vi "FTS GetSet Acquisition Option WMtr Cycle Counting.vi"(6 "readWrite":enum16{"read", "write"}(ring), 8 "error in":errorcluster, 9 "cycleCounting":bool, 10 "channel index interferogram":u16, 11 "spectrometerIdx":u16) -> (0 "error out":errorcluster, 1 "cycleCounting read":bool, 3 "FTSLib_status":i32)   [LabVIEW 2010, in "FTSLib.lvlib"]
uses:
  FTSLib.lvlib
  FTSLib.dll
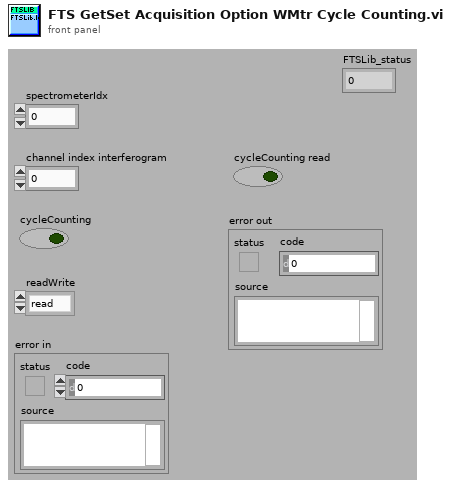
[diagram p1: front panel]
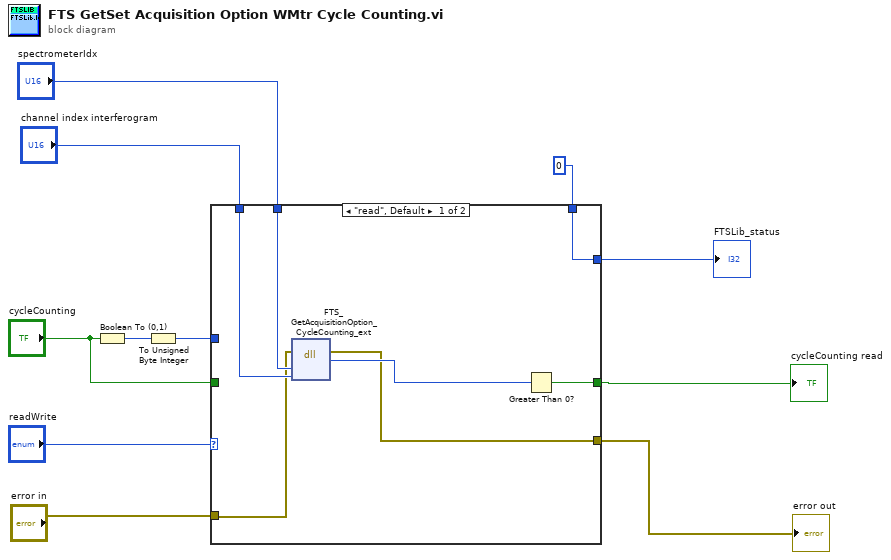
[diagram p0: block diagram]
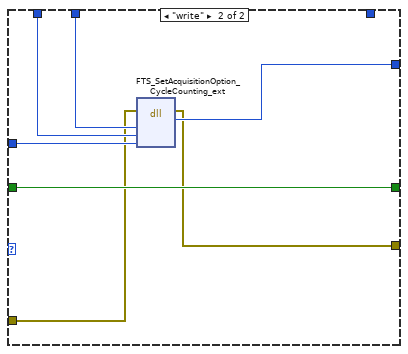
[diagram p2: hidden frame]
diagram:
  n1 = Boolean To (0,1)(Boolean="cycleCounting") -> (0, 1=w6:i16)
  n2 = To Unsigned Byte Integer(number=w6) -> (unsigned 8bit integer=w7:u8)
  n3 = case shown="\"read\", Default" "readWrite" {
    tunnel: "spectrometerIdx" -> [w18 w25]
    tunnel: w7 -> [_ w24]
    tunnel: "error in" -> [w14 w20]
    tunnel: "cycleCounting" -> [_ w23]
    tunnel: [w17 w23] -> w10
    tunnel: [w13 w19] -> w9
    tunnel: "channel index interferogram" -> [w16 w22]
    tunnel: [w12 w21] -> w2
    tunnel: 0 ("return type") -> [w12 _]
    frame "read", Default {
      n4 = dll-call lib="FTSLib.dll" fn="FTS_GetAcquisitionOption_CycleCounting_ext"(error in=w14, "spectrIdx"=w18, "channel"=w16) -> (error out=w13:errorcluster, "return type"=w15:i32)  [unwired: 4 in, 1 out]
      n5 = Greater Than 0?(x=w15) -> (x > 0?=w17:bool)
    }
    frame "write" {
      n6 = dll-call lib="FTSLib.dll" fn="FTS_SetAcquisitionOption_CycleCounting_ext"(error in=w20, "spectrIdx"=w25, "channel"=w22, "cycleCounting"=w24) -> (error out=w19:errorcluster, "return type"=w21:i32)  [unwired: 5 in, 1 out]
    }
  }
  "cycleCounting read" <- w10
  "error out" <- w9
  "FTSLib_status" <- w2
